vi "Heat_Tape_Main.vi"() -> ()   [LabVIEW 2019]
uses:
  Heat_Tape_Global.vi
  <vilib>/NI/Modbus Library/API/Master/Modbus Master.lvclass
  <vilib>/Utility/SystemLogging/NI_SystemLogging.lvlib
panel:
  in  "manual_output_2":bool caption="Manual Output"
  in  "mode_2":enum16{"Auto", "Manual"}(ring) caption="Control Mode"
  in  "test":bool
  in  "mode_1":enum16{"Auto", "Manual"}(ring) caption="Control Mode"
  in  "manual_output_1":bool caption="Manual Output"
  out "curr_1":dbl caption="CH 1" format="%.2f"
  in  "get_curr":bool
  out "curr_2":dbl caption="CH 2" format="%.2f"
  out "ele_pwr_1":dbl caption="CH 1" format="%.1f"
  in  "get_ele_pwr":bool
  out "ele_pwr_2":dbl caption="CH 2" format="%.1f"
  out "status_log":bool caption="Status"
  in  "logging_on":bool caption="Logging"
  out "T_CJ2":dbl caption="CH 2" format="%.1f"
  out "T_CJ1":dbl caption="CH 1" format="%.1f"
  in  "get_CJ_temp":bool
  in  "clear_chart":bool=TRUE caption="Clear charts\nto start"
  out "status_read":bool=TRUE caption="Readout"
  out "chart_t":waveform(dbl)[](graph)=[{"t0"=timestamp(3785686355.130285 s since 1904-01-01), "dt"=1.0, "Y"=[-0.00251999]}, {"t0"=timestamp(3785686355.130285 s since 1904-01-01), "dt"=1.0, "Y"=[-0.00346989]}]
  out "time_meas":timestamp caption="Last Meas. Time" format="%<%Y-%m-%d %H:%M:%S>T"
  in  "SV2_set":dbl=70.5 format="%.1f"
  in  "set_SV2":bool
  out "OUT2":bool
  out "SV2":dbl caption="Set value" format="%.1f"
  out "PV2":dbl caption="Reading" format="%.1f"
  in  "UID2":u8=2
  out "OUT1":bool
  in  "set_SV1":bool
  in  "Interval":i32=1000
  in  "stop":bool
  out "SV1":dbl caption="Set value" format="%.1f"
  out "PV1":dbl caption="Reading" format="%.1f"
  in  "SV1_set":dbl=70.5 format="%.1f"
  in  "UID1":u8=1
  in  "VISA":refnum<visa-resource-name>="COM42"
  # "Heat Tapes for Target Magnet"
  # "Fuji Electronic PXF4"
  # "ms"
  # "CH 1:  IVC"
  # "CH 2:  Turret"
  # "°F"
  # "°F"
  # "°F"
  # "°F"
  # "°F"
  # "°F"
  # "°F"
  # "°F"
  # "W"
  # "W"
  # "A"
  # "A"
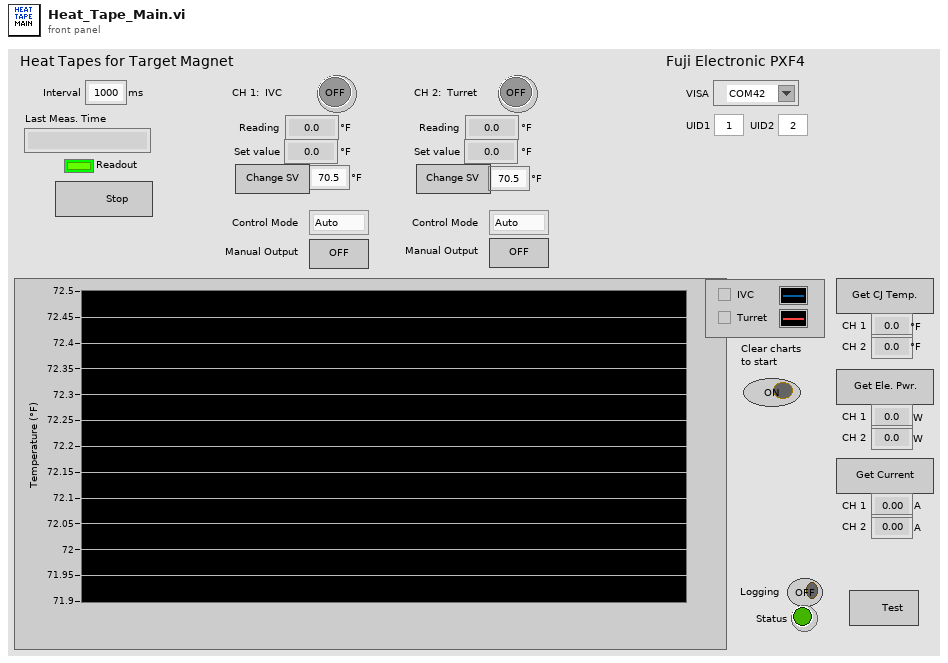
[diagram p1: front panel]
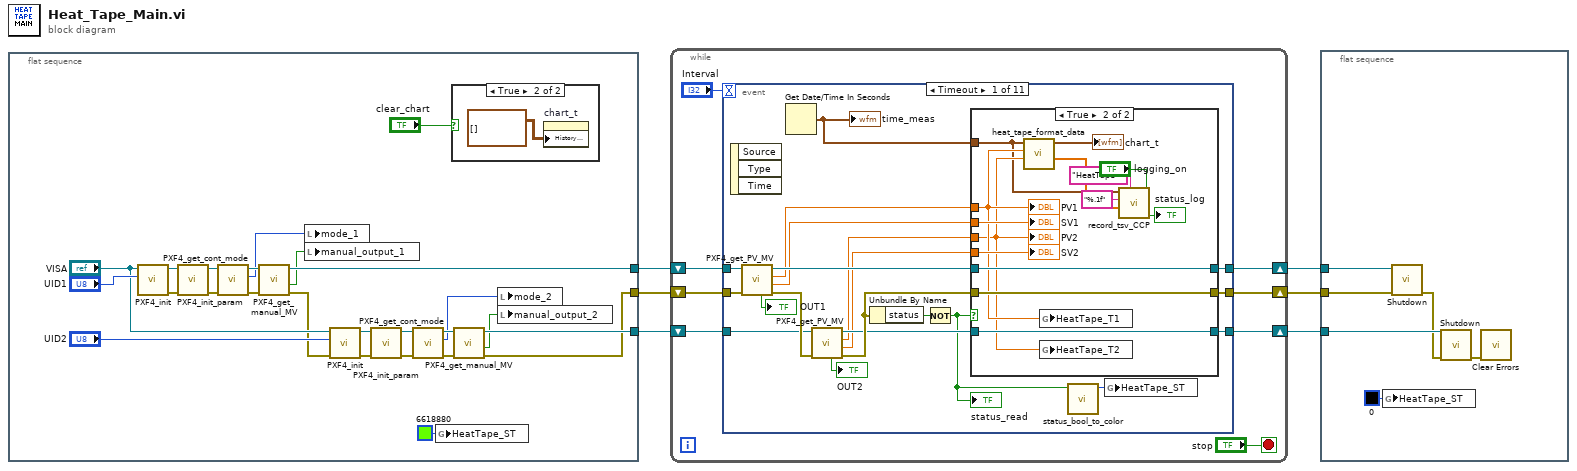
[diagram p0: block diagram]
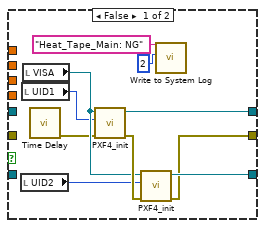
[diagram p3: hidden frame]
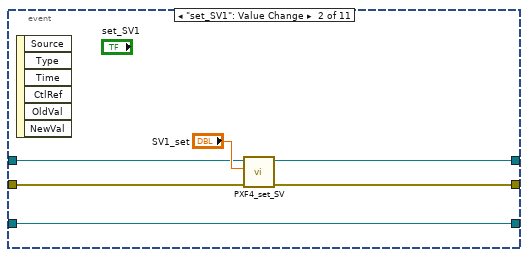
[diagram p4: hidden frame]
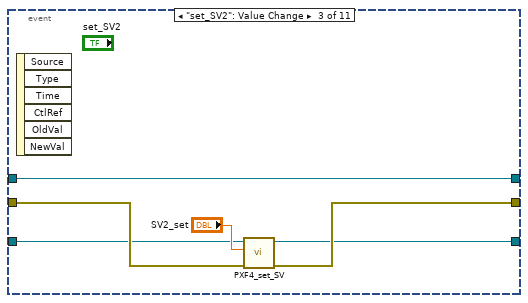
[diagram p5: hidden frame]
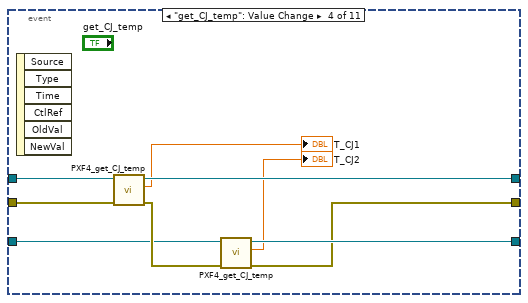
[diagram p6: hidden frame]
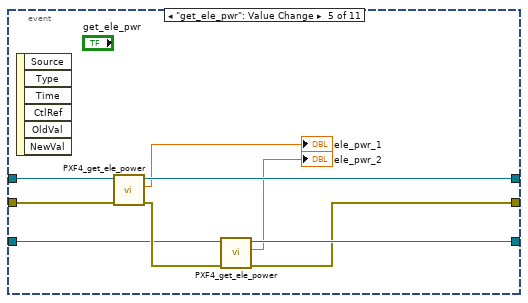
[diagram p7: hidden frame]
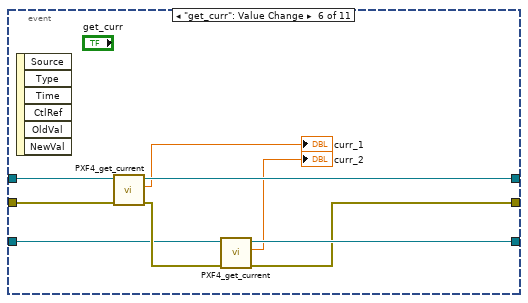
[diagram p8: hidden frame]
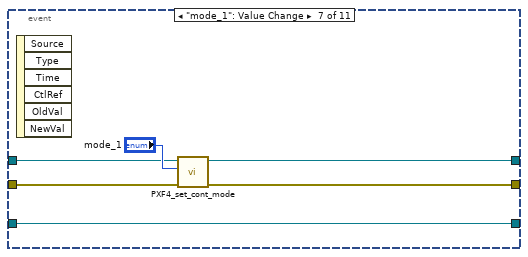
[diagram p9: hidden frame]
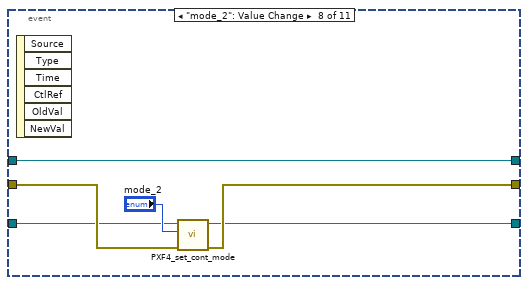
[diagram p10: hidden frame]
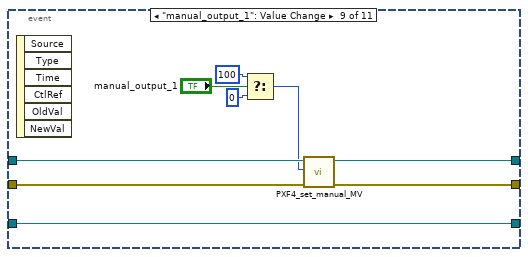
[diagram p11: hidden frame]
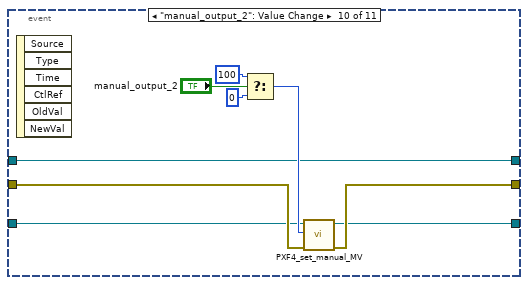
[diagram p12: hidden frame]
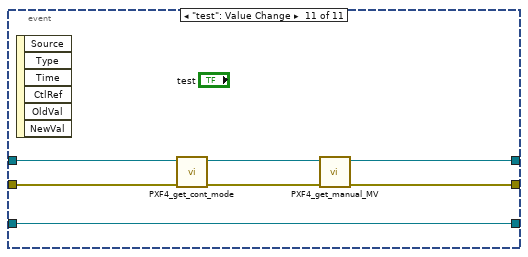
[diagram p13: hidden frame]
diagram:
  n1 = flat-sequence {
    tunnel: [w13] -> w6
    tunnel: [w17] -> w3
    tunnel: [w20] -> w2
    frame #0 {
      n2 = call "PXF4_init.vi"("unit_ID"="UID1", "VISA Refnum in"="VISA") -> ("error out"=w29:errorcluster, "Modbus Master out"=w30:refnum<class "Modbus Master.lvclass">)  [unwired: 8 in]
      n3 = call "PXF4_init_param.vi"("error in"=w29, "Modbus Master in"=w30) -> ("error out"=w11:errorcluster, "Modbus Master out"=w14:refnum<class "Modbus Master.lvclass">)  [unwired: 8 in]
      n4 = call "PXF4_get_cont_mode.vi"("error in"=w11, "Modbus Master in"=w14) -> ("error out"=w15:errorcluster, "mode"=w10:enum16{"Auto", "Manual"}, "Modbus Master out"=w16:refnum<class "Modbus Master.lvclass">)  [unwired: 7 in]
      n5 = call "PXF4_get_manual_MV.vi"("error in"=w15, "Modbus Master in"=w16) -> ("error out"=w12:errorcluster, "onoff"=w9:bool, "Modbus Master out"=w13:refnum<class "Modbus Master.lvclass">)  [unwired: 6 in, 1 out]
      n6 = local write "mode_1"(w10) -> ()
      n7 = local write "manual_output_1"(w9) -> ()
      n8 = call "PXF4_init.vi"("error in"=w12, "unit_ID"="UID2", "VISA Refnum in"="VISA") -> ("error out"=w26:errorcluster, "Modbus Master out"=w28:refnum<class "Modbus Master.lvclass">)  [unwired: 7 in]
      n9 = call "PXF4_init_param.vi"("error in"=w26, "Modbus Master in"=w28) -> ("error out"=w19:errorcluster, "Modbus Master out"=w21:refnum<class "Modbus Master.lvclass">)  [unwired: 8 in]
      n10 = call "PXF4_get_cont_mode.vi"("error in"=w19, "Modbus Master in"=w21) -> ("error out"=w18:errorcluster, "mode"=w8:enum16{"Auto", "Manual"}, "Modbus Master out"=w22:refnum<class "Modbus Master.lvclass">)  [unwired: 7 in]
      n11 = global write "Heat_Tape_Global.vi" "HeatTape_ST"(u32 6618880 ("MKS946_ST")) -> ()
      n12 = case shown="True" "clear_chart" {
        frame False {
        }
        frame True {
          n13 = property on="chart_t" class="WFChart (strict)"("History Data"=waveform(dbl)[][] []) -> ()  [unwired: 2 in, 2 out]
        }
      }
      n14 = call "PXF4_get_manual_MV.vi"("error in"=w18, "Modbus Master in"=w22) -> ("error out"=w17:errorcluster, "onoff"=w7:bool, "Modbus Master out"=w20:refnum<class "Modbus Master.lvclass">)  [unwired: 6 in, 1 out]
      n15 = local write "mode_2"(w8) -> ()
      n16 = local write "manual_output_2"(w7) -> ()
    }
  }
  n17 = while {
    shift-right: [w37] -> w5
    shift-left: w6 -> [w40]
    shift-right: [w38] -> w4
    shift-left: w3 -> [w39]
    shift-right: [w33] -> w1
    shift-left: w2 -> [w34]
    stop <- "stop" stop-if-true
    n18 = event shown="[0] Timeout" {
      selector: _ -> [_ _ _ _ _ _ _ _ _ _ _]
      dyn-events: _ -> [_ _ _ _ _ _ _ _ _ _ _]
      timeout: "Interval" -> [_ _ _ _ _ _ _ _ _ _ _]
      tunnel: w40 -> [w60 w86 w91 w105 w114 w123 w128 w130 w144 w145 w160]
      tunnel: w39 -> [w59 w87 w94 w103 w112 w121 w127 w134 w141 w152 w155]
      tunnel: [w51 w88 w95 w99 w108 w117 w126 w133 w142 w153 w157] -> w38
      tunnel: [w52 w89 w91 w104 w113 w122 w125 w130 w143 w145 w158] -> w37
      tunnel: w34 -> [w56 w85 w93 w101 w110 w119 w124 w132 w140 w147 w154]
      tunnel: [w48 w85 w92 w100 w109 w118 w124 w131 w140 w146 w154] -> w33
      event Timeout {
        n19 = event-data() -> ()  [unwired: 1 in, 3 out]
        n20 = call "PXF4_get_PV_MV.vi"("error in"=w59, "Modbus Master in"=w60) -> ("error out"=w57:errorcluster, "SV"=w45:dbl, "PV"=w44:dbl, "Modbus Master out"=w53:refnum<class "Modbus Master.lvclass">, "Output"=→"OUT1":bool)  [unwired: 5 in]
        n21 = Get Date/Time In Seconds() -> (seconds since 1Jan1904=w41:timestamp)
        "time_meas" <- w41
        n22 = call "PXF4_get_PV_MV.vi"("error in"=w57, "Modbus Master in"=w56) -> ("error out"=w50:errorcluster, "SV"=w47:dbl, "PV"=w46:dbl, "Modbus Master out"=w49:refnum<class "Modbus Master.lvclass">, "Output"=→"OUT2":bool)  [unwired: 5 in]
        n23 = Unbundle By Name(w50) -> ("status"=w54:bool)
        n24 = Not(x=w54) -> (.not. x?=w42:bool)
        "status_read" <- w42
        n25 = case shown="True" w42 {
          tunnel: w53 -> [_ w84]
          tunnel: [w70 w84] -> w52
          tunnel: [w67 w83] -> w51
          tunnel: w50 -> [_ w83]
          tunnel: w49 -> [_ w82]
          tunnel: [w69 w82] -> w48
          tunnel: w47 -> [_ w81]
          tunnel: w46 -> [_ w77]
          tunnel: w45 -> [_ w80]
          tunnel: w44 -> [_ w78]
          tunnel: w41 -> [_ w75]
          frame False {
            n26 = local read "UID2"() -> (w63:u8)
            n27 = local read "UID1"() -> (w64:u8)
            n28 = local read "VISA"() -> (w66:refnum<visa-resource-name>)
            n29 = call "Time Delay"() -> ("error out"=w65:errorcluster)  [unwired: 11 in]
            n30 = call "PXF4_init.vi"("error in"=w65, "unit_ID"=w64, "VISA Refnum in"=w66) -> ("error out"=w68:errorcluster, "Modbus Master out"=w70:refnum<class "Modbus Master.lvclass">)  [unwired: 7 in]
            n31 = call "PXF4_init.vi"("error in"=w68, "unit_ID"=w63, "VISA Refnum in"=w66) -> ("error out"=w67:errorcluster, "Modbus Master out"=w69:refnum<class "Modbus Master.lvclass">)  [unwired: 7 in]
            n32 = call <vilib>:"Write to System Log.vi"("severity"=2, "message"="Heat_Tape_Main: NG") -> ()  [unwired: 9 in, 1 out]
          }
          frame True {
            n33 = call "heat_tape_format_data.vi"("t2"=w77, "t1"=w78, "time"=w75) -> ("t_array"=w76:dbl[], "waveform_array"=→"chart_t":waveform(dbl)[])  [unwired: 7 in]
            n34 = global write "Heat_Tape_Global.vi" "HeatTape_T1"(w78) -> ()
            n35 = global write "Heat_Tape_Global.vi" "HeatTape_T2"(w77) -> ()
            n36 = call "record_tsv_CCP.vi"("logging_on"="logging_on", "folder_name"="HeatTape", "value_array"=w76, "format"="%.1f", "time"=w75) -> ("status_log"=→"status_log":bool)  [unwired: 5 in, 1 out]
            "PV1" <- w78
            "SV1" <- w80
            "PV2" <- w77
            "SV2" <- w81
          }
        }
        n37 = call "status_bool_to_color.vi"("status_bool_1"=w42) -> ("status_color"=w43:u32)  [unwired: 10 in]
        n38 = global write "Heat_Tape_Global.vi" "HeatTape_ST"(w43) -> ()
      }
      event "set_SV1": Value Change {
        n39 = event-data() -> ()  [unwired: 1 in, 6 out]
        n40 = call "PXF4_set_SV.vi"("error in"=w87, "SV"="SV1_set", "Modbus Master in"=w86) -> ("error out"=w88:errorcluster, "Modbus Master out"=w89:refnum<class "Modbus Master.lvclass">)  [unwired: 7 in]
      }
      event "set_SV2": Value Change {
        n41 = event-data() -> ()  [unwired: 1 in, 6 out]
        n42 = call "PXF4_set_SV.vi"("error in"=w94, "SV"="SV2_set", "Modbus Master in"=w93) -> ("error out"=w95:errorcluster, "Modbus Master out"=w92:refnum<class "Modbus Master.lvclass">)  [unwired: 7 in]
      }
      event "get_CJ_temp": Value Change {
        n43 = event-data() -> ()  [unwired: 1 in, 6 out]
        n44 = call "PXF4_get_CJ_temp.vi"("error in"=w103, "Modbus Master in"=w105) -> ("error out"=w102:errorcluster, "degF"=→"T_CJ1":dbl, "Modbus Master out"=w104:refnum<class "Modbus Master.lvclass">)  [unwired: 7 in]
        n45 = call "PXF4_get_CJ_temp.vi"("error in"=w102, "Modbus Master in"=w101) -> ("error out"=w99:errorcluster, "degF"=→"T_CJ2":dbl, "Modbus Master out"=w100:refnum<class "Modbus Master.lvclass">)  [unwired: 7 in]
      }
      event "get_ele_pwr": Value Change {
        n46 = event-data() -> ()  [unwired: 1 in, 6 out]
        n47 = call "PXF4_get_ele_power.vi"("error in"=w112, "Modbus Master in"=w114) -> ("error out"=w111:errorcluster, "W"=→"ele_pwr_1":dbl, "Modbus Master out"=w113:refnum<class "Modbus Master.lvclass">)  [unwired: 7 in]
        n48 = call "PXF4_get_ele_power.vi"("error in"=w111, "Modbus Master in"=w110) -> ("error out"=w108:errorcluster, "W"=→"ele_pwr_2":dbl, "Modbus Master out"=w109:refnum<class "Modbus Master.lvclass">)  [unwired: 7 in]
      }
      event "get_curr": Value Change {
        n49 = event-data() -> ()  [unwired: 1 in, 6 out]
        n50 = call "PXF4_get_current.vi"("error in"=w121, "Modbus Master in"=w123) -> ("error out"=w120:errorcluster, "A"=→"curr_1":dbl, "Modbus Master out"=w122:refnum<class "Modbus Master.lvclass">)  [unwired: 7 in]
        n51 = call "PXF4_get_current.vi"("error in"=w120, "Modbus Master in"=w119) -> ("error out"=w117:errorcluster, "A"=→"curr_2":dbl, "Modbus Master out"=w118:refnum<class "Modbus Master.lvclass">)  [unwired: 7 in]
      }
      event "mode_1": Value Change {
        n52 = event-data() -> ()  [unwired: 1 in, 6 out]
        n53 = call "PXF4_set_cont_mode.vi"("error in"=w127, "mode"="mode_1", "Modbus Master in"=w128) -> ("error out"=w126:errorcluster, "Modbus Master out"=w125:refnum<class "Modbus Master.lvclass">)  [unwired: 7 in]
      }
      event "mode_2": Value Change {
        n54 = event-data() -> ()  [unwired: 1 in, 6 out]
        n55 = call "PXF4_set_cont_mode.vi"("error in"=w134, "mode"="mode_2", "Modbus Master in"=w132) -> ("error out"=w133:errorcluster, "Modbus Master out"=w131:refnum<class "Modbus Master.lvclass">)  [unwired: 7 in]
      }
      event "manual_output_1": Value Change {
        n56 = event-data() -> ()  [unwired: 1 in, 6 out]
        n57 = Select(t=u8 100, s="manual_output_1", f=u8 0) -> (s? t:f=w136:u8)
        n58 = call "PXF4_set_manual_MV.vi"("error in"=w141, "MV_manual"=w136, "Modbus Master in"=w144) -> ("error out"=w142:errorcluster, "Modbus Master out"=w143:refnum<class "Modbus Master.lvclass">)  [unwired: 7 in]
      }
      event "manual_output_2": Value Change {
        n59 = event-data() -> ()  [unwired: 1 in, 6 out]
        n60 = Select(t=u8 100, s="manual_output_2", f=u8 0) -> (s? t:f=w148:u8)
        n61 = call "PXF4_set_manual_MV.vi"("error in"=w152, "MV_manual"=w148, "Modbus Master in"=w147) -> ("error out"=w153:errorcluster, "Modbus Master out"=w146:refnum<class "Modbus Master.lvclass">)  [unwired: 7 in]
      }
      event "test": Value Change {
        n62 = event-data() -> ()  [unwired: 1 in, 6 out]
        n63 = call "PXF4_get_cont_mode.vi"("error in"=w155, "Modbus Master in"=w160) -> ("error out"=w156:errorcluster, "Modbus Master out"=w159:refnum<class "Modbus Master.lvclass">)  [unwired: 7 in, 1 out]
        n64 = call "PXF4_get_manual_MV.vi"("error in"=w156, "Modbus Master in"=w159) -> ("error out"=w157:errorcluster, "Modbus Master out"=w158:refnum<class "Modbus Master.lvclass">)  [unwired: 6 in, 2 out]
      }
    }
  }
  n65 = flat-sequence {
    tunnel: w5 -> [w166]
    tunnel: w4 -> [w165]
    tunnel: w1 -> [w164]
    frame #0 {
      n66 = global write "Heat_Tape_Global.vi" "HeatTape_ST"(u32 0 ("MKS946_ST")) -> ()
      n67 = call-dynamic "Shutdown.vi"("error in"=w165, "Modbus master in"=w166) -> ("error out"=w163:errorcluster)  [unwired: 9 in]
      n68 = call-dynamic "Shutdown.vi"("error in"=w163, "Modbus master in"=w164) -> ("error out"=w162:errorcluster)  [unwired: 9 in]
      n69 = call <vilib>:"Clear Errors.vi"("error in (no error)"=w162) -> ()  [unwired: 5 in, 2 out]
    }
  }
